vi "Read last shots from log.vi"(8 "Error In":errorcluster, 10 "tail length to read":i64=512, 11 "Shots file":path=path "Z:/ShotHistory2014.txt") -> (0 "Error Out":errorcluster, 1 "Tail string":string, 2 "Last shots strings":string[](array[string]), 3 "Last shots":T1[](array[typedef]))   [LabVIEW 2015]
uses:
  Shot data.ctl
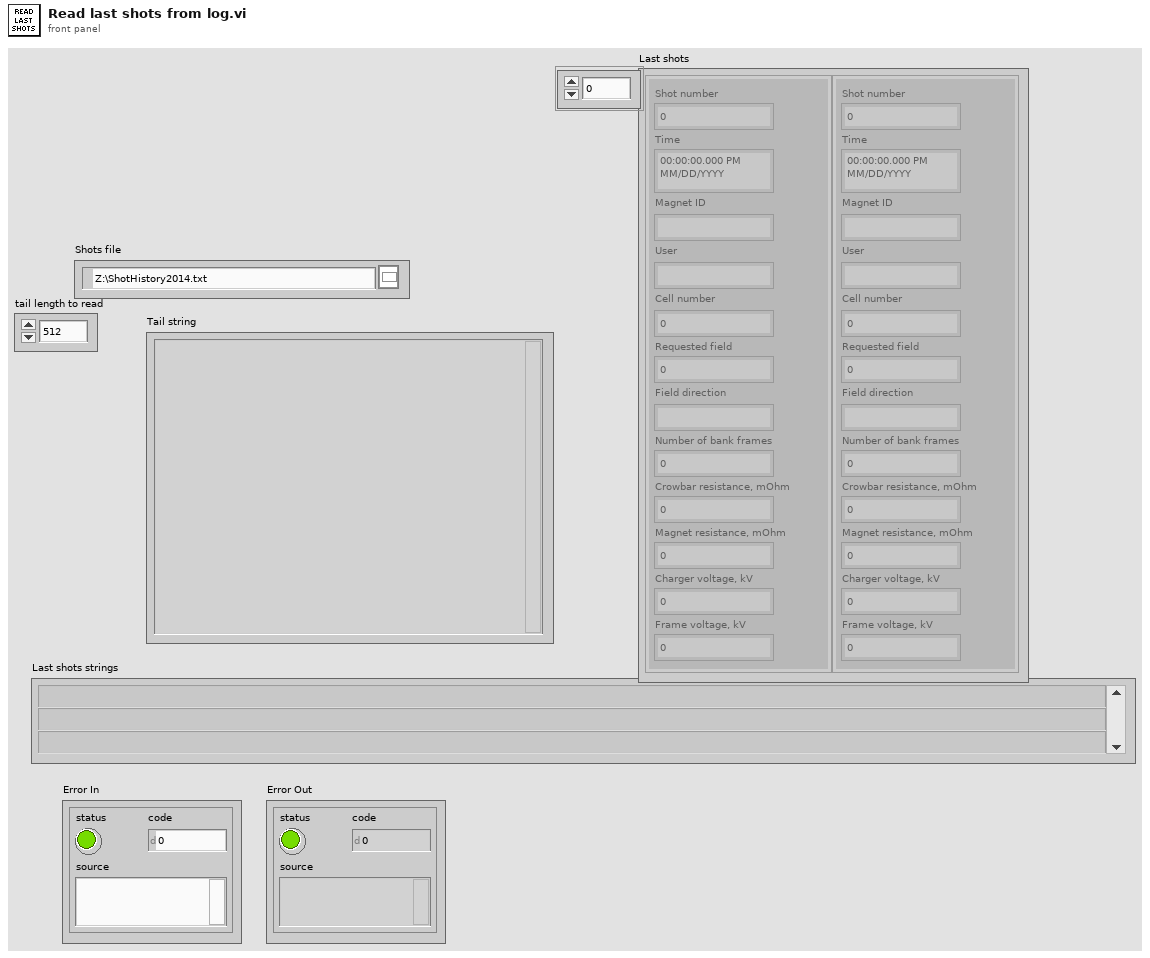
[diagram p1: front panel]
types:
  T1 = typedef "Shot data.ctl" = cluster{"Shot number":i32, "Time":timestamp, "Magnet ID":string, "User":string, "Cell number":i32, "Requested field":dbl, "Field direction":string, "Number of bank frames":i32, "Crowbar resistance, mOhm":dbl, "Magnet resistance, mOhm":dbl, "Charger voltage, kV":dbl, "Frame voltage, kV":dbl}
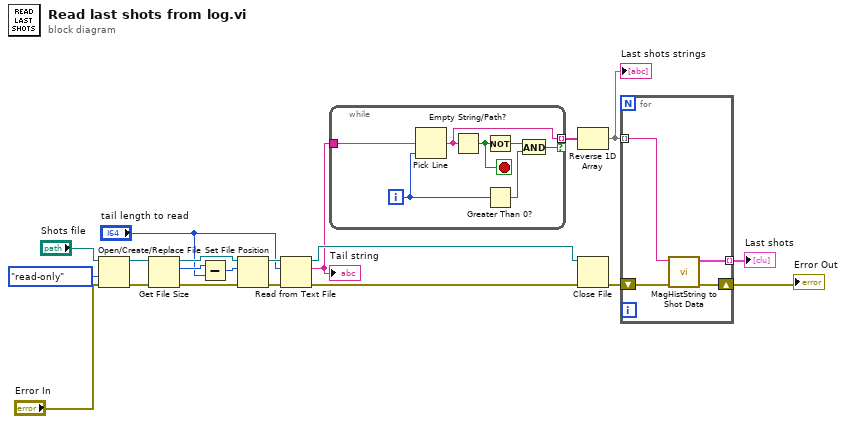
[diagram p0: block diagram]
diagram:
  n1 = Open/Create/Replace File(file path (use dialog)="Shots file", error in="Error In", access (0:read/write)=enum16{"read/write", "read-only", "write-only"}."read-only") -> (refnum out=w18:refnum<file>, error out=w19:errorcluster)  [unwired: 3 in, 1 out]
  n2 = Get File Size(file=w18, error in=w19) -> (refnum out=w16:refnum<file>, size (in bytes)=w15:i64, 0:w17:errorcluster)
  n3 = Subtract(x=w15, y="tail length to read") -> (x-y=w14:i64)
  n4 = Set File Position(offset (in bytes) (0)=w14, refnum=w16, error in=w17) -> (refnum out=w12:refnum<file>, error out=w13:errorcluster)  [unwired: 1 in]
  n5 = Read from Text File(file (use dialog)=w12, count="tail length to read", error in=w13) -> (refnum out=w9:refnum<file>, text=w7:string, error out=w10:errorcluster)  [unwired: 1 in, 1 out]
  "Tail string" <- w7
  n6 = while {
    tunnel: w7 -> [w27]
    tunnel: [w22] -> w6 mode=indexing if=w21
    i -> [w26]
    stop <- w25 stop-if-true
    n7 = Pick Line(multi-line string=w27, line index=w26) -> (output string=w22:string)  [unwired: 1 in]
    n8 = Empty String/Path?(string/path=w22) -> (empty?=w25:bool)
    n9 = Not(x=w25) -> (.not. x?=w23:bool)
    n10 = Greater Than 0?(x=w26) -> (x > 0?=w24:bool)
    n11 = And(x=w23, y=w24) -> (x .and. y?=w21:bool)
  }
  n12 = Reverse 1D Array(array=w6) -> (reversed array=w3:string[])
  "Last shots strings" <- w3
  n13 = Close File(refnum=w9, error in=w10) -> (error out=w4:errorcluster)  [unwired: 1 out]
  n14 = for {
    tunnel: w3 -> [w31] mode=indexing
    tunnel: [w30] -> w5 mode=indexing
    shift-right: [w28] -> w2
    shift-left: w4 -> [w29]
    n15 = call "MagHistString to Shot Data.vi"("error in (no error)"=w29, "String"=w31) -> ("error out"=w28:errorcluster, "Shot data"=w30:T1)  [unwired: 8 in]
  }
  "Last shots" <- w5
  "Error Out" <- w2
